vi "_CH375_Set.vi"(8 "Error In":errorcluster, 10 "设定角度":dbl, 11 "移动速度":u16(ring)=1 items=["1", "1/2", "1/4", "1/8", "1/16", "1/32", "1/64", "1/128"]) -> (0 "Error Out":errorcluster, 3 "设置成功":bool=TRUE)   [LabVIEW 2020, in "CH375.lvlib"]
uses:
  CH375.lvlib
  CH375DLL64.dll
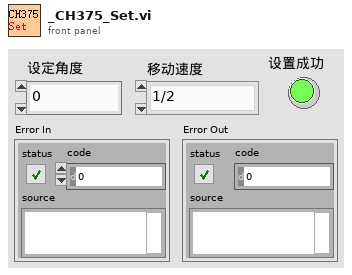
[diagram p1: front panel]
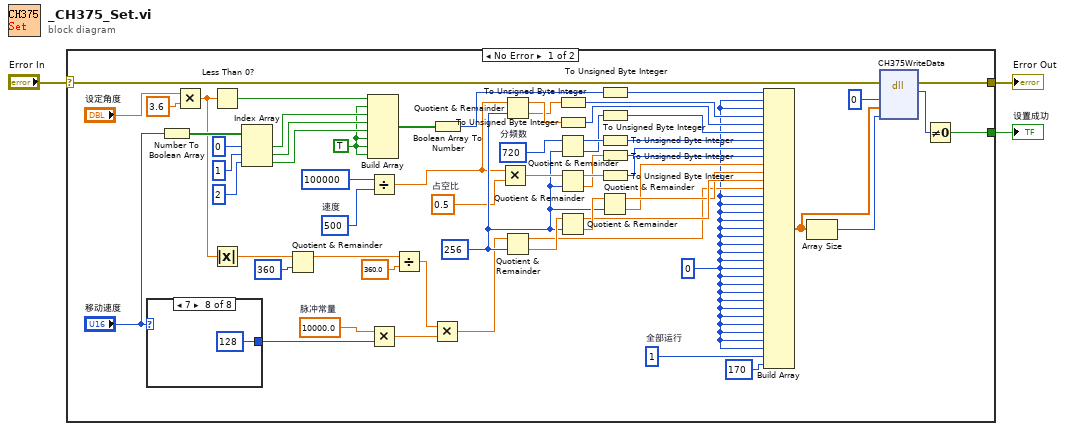
[diagram p0: block diagram]
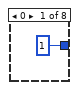
[diagram p2: hidden frame]
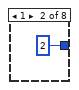
[diagram p3: hidden frame]
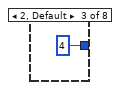
[diagram p4: hidden frame]
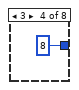
[diagram p5: hidden frame]
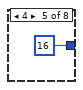
[diagram p6: hidden frame]
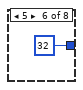
[diagram p7: hidden frame]
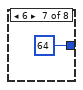
[diagram p8: hidden frame]
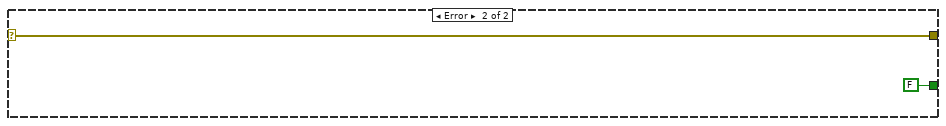
[diagram p9: hidden frame]
diagram:
  n1 = case shown="No Error" "Error In" {
    selector: "Error In" -> [w63 w73]
    tunnel: [w62 w73] -> w2
    tunnel: [w61 FALSE] -> w1
    frame No Error {
      w9 = 10000.0  # 脉冲常量
      w13 = 1  # 全部运行
      w15 = 0.5  # 占空比
      w16 = 720  # 分频数
      w17 = 500  # 速度
      w23 = 0 ("element")
      w14 = TRUE ("元素")
      w47 = u16 256 ("y")
      n2 = case shown="7" "移动速度" {
        tunnel: [1 2 4 8 16 32 64 128] -> w12
        frame 0 {
        }
        frame 1 {
        }
        frame 2, Default {
        }
        frame 3 {
        }
        frame 4 {
        }
        frame 5 {
        }
        frame 6 {
        }
        frame 7 {
        }
      }
      n3 = Number To Boolean Array(number="移动速度") -> (Boolean array=w44:bool[])
      n4 = Multiply(x="设定角度", y=3.6) -> (x*y=w10:dbl)
      n5 = Less Than 0?(x=w10) -> (x < 0?=w7:bool)
      n6 = Absolute Value(x=w10) -> (abs(x)=w6:dbl)
      n7 = Index Array(array=w44, index #1=0 ("索引"), index #2=1 ("索引"), index #3=2 ("索引")) -> (element #1=w40:bool, element #2=w39:bool, element #3=w38:bool)
      n8 = Quotient & Remainder(x=w6, y=360) -> (x-y*floor(x/y)=w5:dbl)  [unwired: 1 out]
      n9 = Build Array(w7, w14, w40, w39, w38, w14, w14, w14) -> (w46:bool[])
      n10 = Divide(x=u32 100000, y=w17) -> (x/y=w25:dbl)
      n11 = Multiply(x=w9, y=w12) -> (x*y=w18:dbl)
      n12 = Divide(x=w5, y=360.0) -> (x/y=w22:dbl)
      n13 = Multiply(x=w22, y=w18) -> (x*y=w21:dbl)
      n14 = Boolean Array To Number(Boolean array=w46) -> (number=w45:u32)
      n15 = Multiply(x=w25, y=w15) -> (x*y=w50:dbl)
      n16 = Quotient & Remainder(x=w25, y=w47) -> (x-y*floor(x/y)=w56:dbl, floor(x/y)=w55:dbl)
      n17 = Quotient & Remainder(x=w21, y=w47) -> (x-y*floor(x/y)=w26:dbl, floor(x/y)=w49:dbl)
      n18 = To Unsigned Byte Integer(number=w55) -> (unsigned 8bit integer=w28:u8)
      n19 = To Unsigned Byte Integer(number=w56) -> (unsigned 8bit integer=w29:u8)
      n20 = Quotient & Remainder(x=w16, y=w47) -> (x-y*floor(x/y)=w54:i32, floor(x/y)=w53:i32)
      n21 = Quotient & Remainder(x=w50, y=w47) -> (x-y*floor(x/y)=w52:dbl, floor(x/y)=w51:dbl)
      n22 = Quotient & Remainder(x=w49, y=w47) -> (x-y*floor(x/y)=w36:dbl, floor(x/y)=w48:dbl)
      n23 = To Unsigned Byte Integer(number=w45) -> (unsigned 8bit integer=w37:u8)
      n24 = To Unsigned Byte Integer(number=w53) -> (unsigned 8bit integer=w30:u8)
      n25 = To Unsigned Byte Integer(number=w54) -> (unsigned 8bit integer=w31:u8)
      n26 = To Unsigned Byte Integer(number=w51) -> (unsigned 8bit integer=w32:u8)
      n27 = To Unsigned Byte Integer(number=w52) -> (unsigned 8bit integer=w33:u8)
      n28 = Quotient & Remainder(x=w48, y=w47) -> (x-y*floor(x/y)=w35:dbl, floor(x/y)=w34:dbl)
      n29 = Build Array(w37, w23, w23, w28, w29, w30, w31, w32, w33, w34, w35, w36, w26, w23, w23, w23, w23, w23, w23, w23, w23, w23, w23, w23, w23, w23, w23, w23, w23, w23, w23, w23, w23, w13, 170 ("元素")) -> (w60:dbl[])
      n30 = Array Size(array=w60) -> (size(s)=w59:i32)
      n31 = dll-call lib="D:/Project NJU/lib/CH375/CH375DLL64.dll" fn="CH375WriteData"(error in=w63, "iIndex"=u8 0, "oBuffer"=w60, "ioLength"=w59) -> (error out=w62:errorcluster, "返回类型"=w57:i32)  [unwired: 4 in, 2 out]
      n32 = Not Equal To 0?(x=w57) -> (x != 0?=w61:bool)
    }
    frame Error {
    }
  }
  "Error Out" <- w2
  "设置成功" <- w1
